vi "ChangeRightSubpanel.vi"(8 "error in (no error)":errorcluster, 10 "Left Active":i32, 11 "MAUI in":refnum<class "MAUI.lvclass">) -> (0 "error out":errorcluster, 3 "MAUI out":refnum<class "MAUI.lvclass">)   [LabVIEW 2016, in "MAUI.lvclass"]
uses:
  MAUI.lvclass
  MAUI.lvclass/MAUI.ctl
  <vilib>/Levylab/Embedded SMO UI/EmbeddedSMO.lvclass
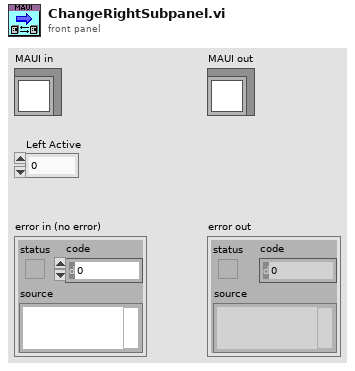
[diagram p1: front panel]
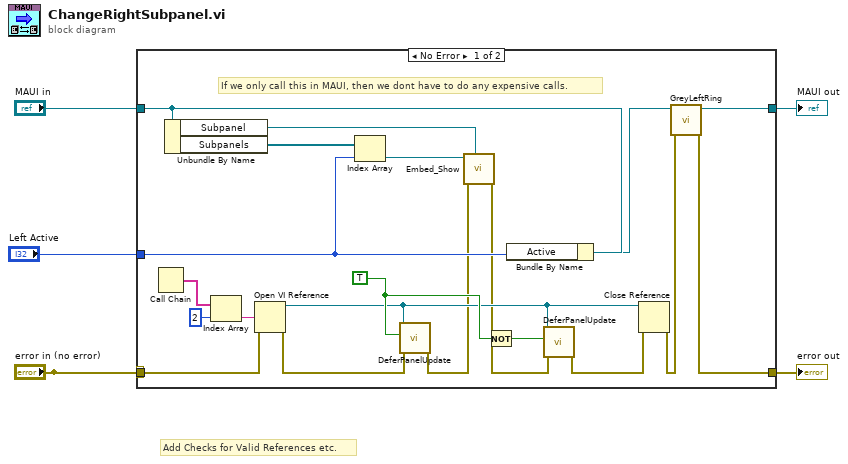
[diagram p0: block diagram]
diagram:
  # "Add Checks for Valid References etc."
  n1 = case shown="No Error" "error in (no error)" {
    selector: "error in (no error)" -> [_ w27]
    tunnel: [w8 w27] -> w5
    tunnel: [w21 w26] -> w3
    tunnel: "MAUI in" -> [w23 w26]
    tunnel: "Left Active" -> [w25 _]
    tunnel: "error in (no error)" -> [w13 _]
    frame No Error {
      w15 = TRUE ("Defer Panel Updates")
      # "If we only call this in MAUI, then we dont have to do any expensive calls."
      n2 = Call Chain() -> (call chain=w6:string[])
      n3 = Unbundle By Name(w23) -> ("Subpanel"=w17:refnum<vi>, "Subpanels"=w24:refnum<class "EmbeddedSMO.lvclass">[])
      n4 = Index Array(array=w6, index=2) -> (element=w19:string)
      n5 = Open VI Reference(vi path=w19, error in (no error)=w13) -> (vi reference=w14:refnum<vi>, error out=w12:errorcluster)  [unwired: 4 in]
      n6 = Index Array(array=w24, index=w25) -> (element=w18:refnum<class "EmbeddedSMO.lvclass">)
      n7 = call <vilib>:"DeferPanelUpdate.vi"("error in (no error)"=w12, "Defer Panel Updates"=w15, "VI in"=w14) -> ("error out"=w11:errorcluster)  [unwired: 8 in]
      n8 = call <vilib>:"Embed_Show.vi"("Sub Panel"=w17, "error in (no error)"=w11, "EmbeddedSMO in"=w18) -> ("error out"=w10:errorcluster)  [unwired: 7 in, 1 out]
      n9 = Not(x=w15) -> (.not. x?=w16:bool)
      n10 = Bundle By Name(cluster=w23, "Active"=w25) -> (w22:refnum<class "MAUI.lvclass">)
      n11 = call <vilib>:"DeferPanelUpdate.vi"("error in (no error)"=w10, "Defer Panel Updates"=w16, "VI in"=w14) -> ("error out"=w9:errorcluster)  [unwired: 8 in]
      n12 = Close Reference(reference=w14, error in (no error)=w9) -> (error out=w7:errorcluster)
      n13 = call "GreyLeftRing.vi"("error in (no error)"=w7, "MAUI in"=w22) -> ("error out"=w8:errorcluster, "MAUI out"=w21:refnum<class "MAUI.lvclass">)  [unwired: 8 in]
    }
    frame Error {
    }
  }
  "error out" <- w5
  "MAUI out" <- w3
